vi "SendNotification.vi"(0 "notification":string, 1 "s":string) -> ()   [LabVIEW 2011]
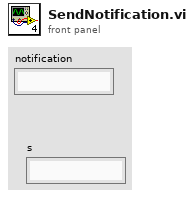
[diagram p1: front panel]
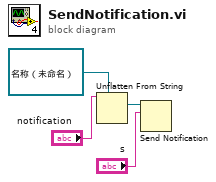
[diagram p0: block diagram]
diagram:
  n1 = Unflatten From String(type=refnum<notifier> refnum ("通知器输出"), binary string="notification") -> (value=w1:refnum<notifier>)  [unwired: 3 in, 2 out]
  n2 = Send Notification(notification="s", notifier=w1) -> ()  [unwired: 1 in, 2 out]
